vi "Experiment_Init.vi"(0 "object in":refnum<class "Experiment.lvclass">, 2 "Cluster":T1, 3 "File Path Control":path, 5 "error in (no error)":errorcluster) -> (14 "object out":refnum<class "Experiment.lvclass">, 19 "error out":errorcluster)   [LabVIEW 2019, in "Experiment.lvclass"]
uses:
  Experiment.lvclass
  AD2_WFG_SDK_class/WFG.ctl
  AD2_WFG_SDK_class/WFGCh.ctl
  AD2_WFG_SDK_class/AD2TriggerSources.ctl
  Experiment.lvclass/Experiment.ctl
  AD2_SDK_class/AD2_SDK.lvclass
  AD2_WFG_SDK_class/AD2_WFG_SDK.lvclass
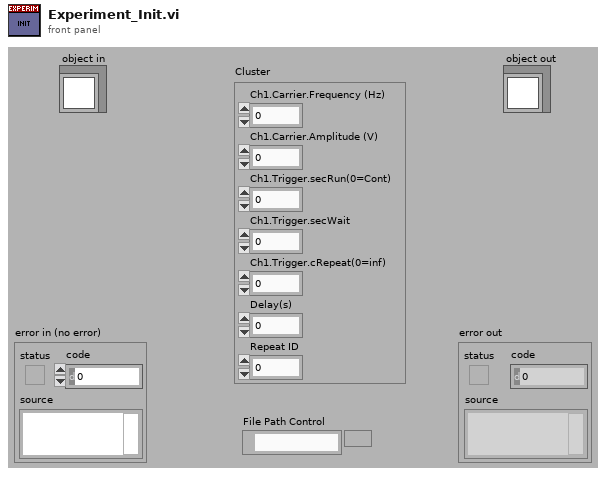
[diagram p1: front panel]
types:
  T1 = cluster{"Ch1.Carrier.Frequency (Hz)":dbl, "Ch1.Carrier.Amplitude (V)":dbl, "Ch1.Trigger.secRun(0=Cont)":dbl, "Ch1.Trigger.secWait":dbl, "Ch1.Trigger.cRepeat(0=inf)":i32, "Delay(s)":dbl, "Repeat ID":i32}
  T2 = typedef "AD2_WFG_SDK.lvclass/WFG.ctl" = cluster{"Running":bool, "Ch1":T3, "Ch2":T3, "SyncronizeState":enum16{"Independent", "Ch1Master", "Ch2Master"}}
  T3 = typedef "AD2_WFG_SDK.lvclass/WFGCh.ctl" = cluster{"idxChannel":i32, "Settings out of range":bool, "Carrier":cluster{"Frequency (Hz)":dbl, "Amplitude (V)":dbl, "Offset(V)":dbl, "Symmetry(%) ":dbl, "Phase(Deg)":dbl, "Function":u16, "Enable":bool}, "Trigger":cluster{"secRun(0=Cont)":dbl, "secWait":dbl, "cRepeat(0=inf)":i32, "Repeat Trigger":bool, "TrigrSrc":T4}, "FM Mod":cluster{"Frequency (Hz)":dbl, "Amplitude (%)":dbl, "Offset(V)":dbl, "Symmetry(%) ":dbl, "Phase(Deg)":dbl, "Function 2":u16, "Enable":bool}}
  T4 = typedef "AD2_SDK.lvclass/AD2TriggerSources.ctl" = enum8{"trigrsrcNone", "trigsrcPC", "trigsrcDetectorAnalogIn", "trigsrcDetectorDigitalIn", "trigsrcAnalogIn", "trigsrcDigitalIn", "trigsrcDigitalOut", "trigsrcAnalogOut1", "trigsrcAnalogOut2", "trigsrcAnalogOut3", "trigsrcAnalogOut4", "trigsrcExternal1", "trigsrcExternal2", "trigsrcExternal3", "trigsrcExternal4", ""}
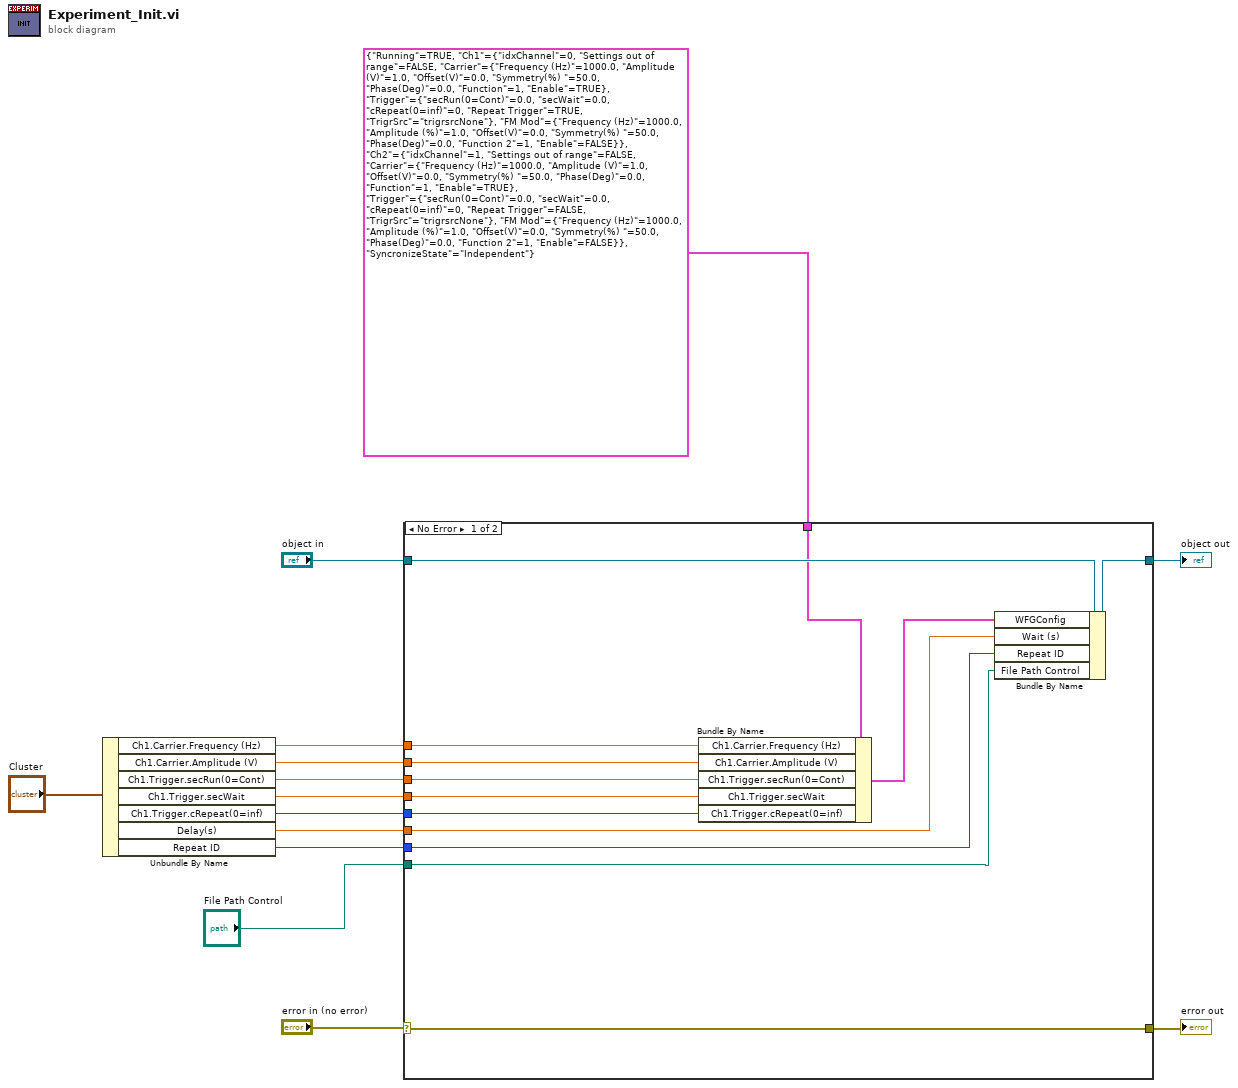
[diagram p0: block diagram]
diagram:
  n1 = Unbundle By Name("Cluster") -> ("Ch1.Carrier.Frequency (Hz)"=w8:dbl, "Ch1.Carrier.Amplitude (V)"=w7:dbl, "Ch1.Trigger.secRun(0=Cont)"=w6:dbl, "Ch1.Trigger.secWait"=w5:dbl, "Ch1.Trigger.cRepeat(0=inf)"=w4:i32, "Delay(s)"=w3:dbl, "Repeat ID"=w2:i32)
  n2 = case shown="No Error" "error in (no error)" {
    selector: "error in (no error)" -> [w25 w28]
    tunnel: "object in" -> [w27 w29]
    tunnel: [w26 w29] -> w13
    tunnel: [w25 w28] -> w11
    tunnel: T2 {"Running"=TRUE, "Ch1"={"idxChannel"=0, "Settings out of range"=FALSE, "Carrier"={"Frequency (Hz)"=1000.0, "Amplitude (V)"=1.0, "Offset(V)"=0.0, "Symmetry(%) "=50.0, "Phase(Deg)"=0.0, "Function"=1, "Enable"=TRUE}, "Trigger"={"secRun(0=Cont)"=0.0, "secWait"=0.0, "cRepeat(0=inf)"=0, "Repeat Trigger"=TRUE, "TrigrSrc"=enum."trigrsrcNone"}, "FM Mod"={"Frequency (Hz)"=1000.0, "Amplitude (%)"=1.0, "Offset(V)"=0.0, "Symmetry(%) "=50.0, "Phase(Deg)"=0.0, "Function 2"=1, "Enable"=FALSE}}, "Ch2"={"idxChannel"=1, "Settings out of range"=FALSE, "Carrier"={"Frequency (Hz)"=1000.0, "Amplitude (V)"=1.0, "Offset(V)"=0.0, "Symmetry(%) "=50.0, "Phase(Deg)"=0.0, "Function"=1, "Enable"=TRUE}, "Trigger"={"secRun(0=Cont)"=0.0, "secWait"=0.0, "cRepeat(0=inf)"=0, "Repeat Trigger"=FALSE, "TrigrSrc"=enum."trigrsrcNone"}, "FM Mod"={"Frequency (Hz)"=1000.0, "Amplitude (%)"=1.0, "Offset(V)"=0.0, "Symmetry(%) "=50.0, "Phase(Deg)"=0.0, "Function 2"=1, "Enable"=FALSE}}, "SyncronizeState"=enum."Independent"} ("WFGConfig") -> [w15 _]
    tunnel: w8 -> [w24 _]
    tunnel: w7 -> [w23 _]
    tunnel: w6 -> [w22 _]
    tunnel: w5 -> [w21 _]
    tunnel: w4 -> [w20 _]
    tunnel: w3 -> [w19 _]
    tunnel: w2 -> [w18 _]
    tunnel: "File Path Control" -> [w17 _]
    frame No Error {
      n3 = Bundle By Name(cluster=w15, "Ch1.Carrier.Frequency (Hz)"=w24, "Ch1.Carrier.Amplitude (V)"=w23, "Ch1.Trigger.secRun(0=Cont)"=w22, "Ch1.Trigger.secWait"=w21, "Ch1.Trigger.cRepeat(0=inf)"=w20) -> (w16:T2)
      n4 = Bundle By Name(cluster=w27, "WFGConfig"=w16, "Wait (s)"=w19, "Repeat ID"=w18, "File Path Control"=w17) -> (w26:refnum<class "Experiment.lvclass">)
    }
    frame Error {
    }
  }
  "object out" <- w13
  "error out" <- w11
